vi "WaitForCMD.vi"(0 "Clients ID IN":refnum<k5>[](array[refnum]), 1 "Cmd FIFO IN":T1(array[cluster]), 5 "TCP/IP Error IN":errorcluster, 9 "Excmd VRN":refnum<visa-resource-name>="COM8", 11 "Serial Error IN":errorcluster, 12 "Timeout":u32=25) -> (3 "Cmd FIFO OUT":T1(array[cluster]), 6 "TCP/IP Error":errorcluster, 15 "Serial Error":errorcluster)   [LabVIEW 2019]
panel:
  out "Chaîne":string
  out "ExecTime":u32
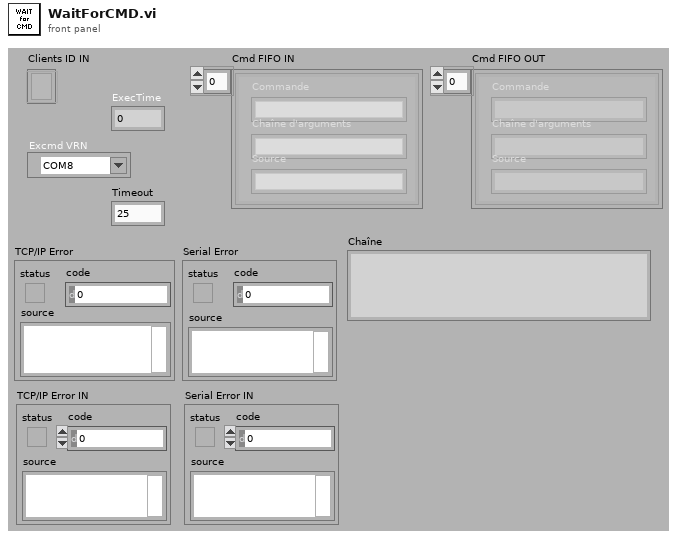
[diagram p1: front panel]
types:
  T1 = cluster{"Commande":string, "Chaîne d'arguments":string, "Source":string}[]
  T2 = cluster{"Commande":string, "data out":string, "Source":string}[]
  T3 = cluster{"Commande":string, "Chaîne":string, "Source":string}[]
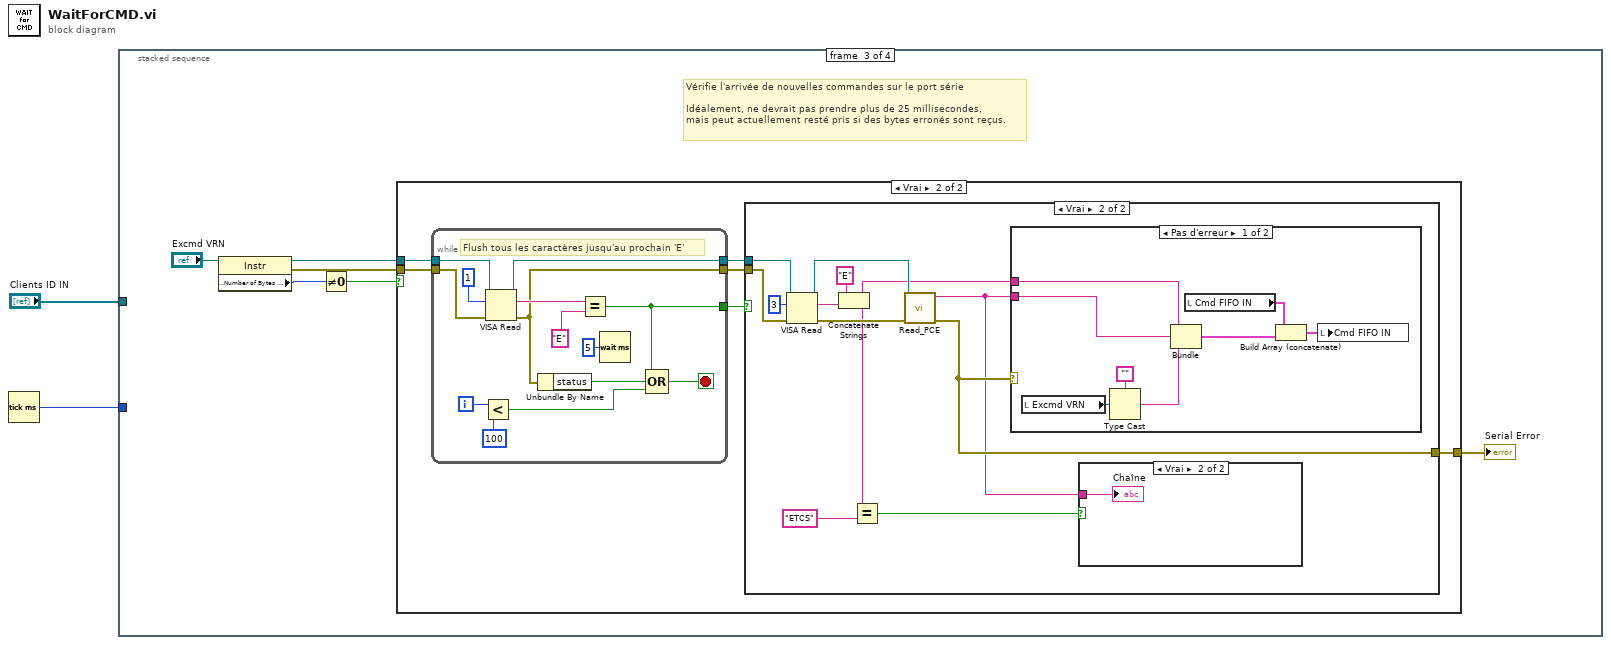
[diagram p0: block diagram]
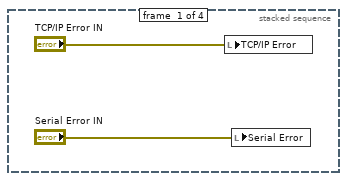
[diagram p2: hidden frame]
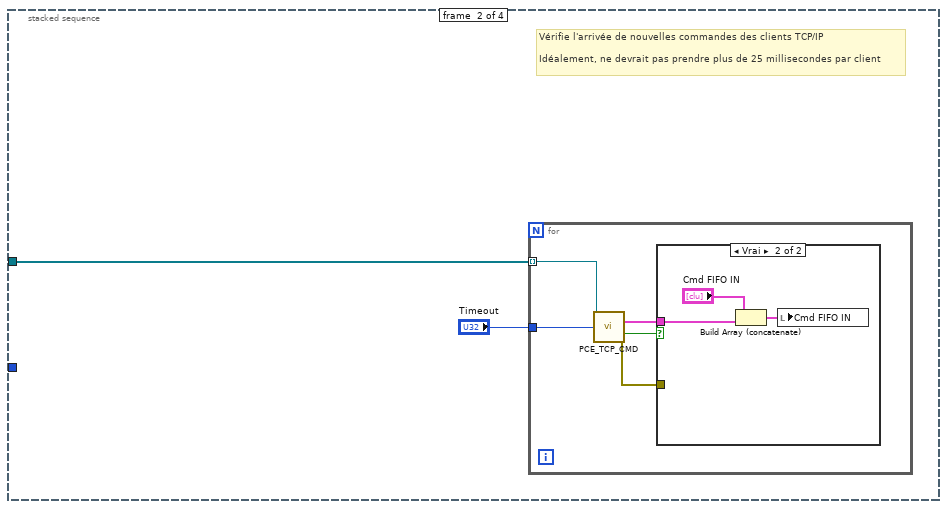
[diagram p3: hidden frame]
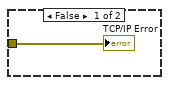
[diagram p4: hidden frame]
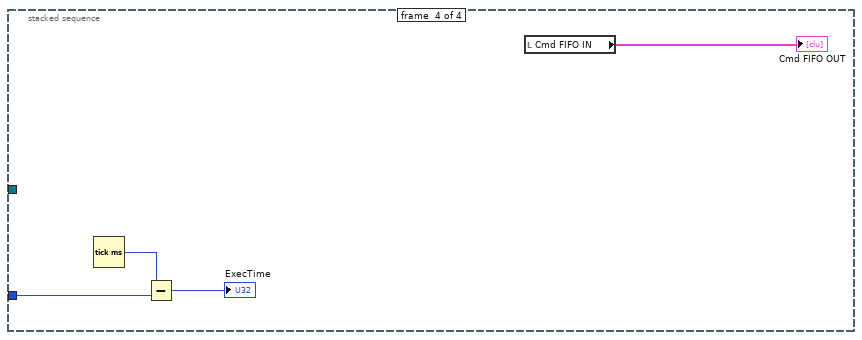
[diagram p9: hidden frame]
diagram:
  n1 = Tick Count (ms)() -> (millisecond timer value=w2:u32)
  n2 = stacked-sequence {
    tunnel: w2 -> [_ _ _ w67]
    tunnel: "Clients ID IN" -> [_ w6 _ _]
    frame #0 {
      n3 = local write "TCP/IP Error"("TCP/IP Error IN") -> ()
      n4 = local write "Serial Error"("Serial Error IN") -> ()
    }
    frame #1 {
      # "Vérifie l'arrivée de nouvelles commandes des clients TCP/IP\n\nIdéalement, ne devrait pas prendre plus de 25 millisecondes par client"
      n5 = for {
        tunnel: w6 -> [w11] mode=indexing
        tunnel: "Timeout" -> [w7]
        n6 = call "PCE_TCP_CMD.vi"("CID IN"=w11, "Timeout"=w7) -> ("FIFOelt"=w9:cluster{string, "data out":string, string}, "Cmd?"=w10:bool, "Error OUT"=w8:errorcluster)  [unwired: 10 in, 1 out]
        n7 = case shown="Vrai" w10 {
          tunnel: w9 -> [_ w14]
          tunnel: w8 -> [w12 _]
          frame False {
            "TCP/IP Error" <- w12
          }
          frame True {
            n8 = Build Array (concatenate)("Cmd FIFO IN", w14) -> (w13:T2)
            n9 = local write "Cmd FIFO IN"(w13) -> ()
          }
        }
      }
    }
    frame #2 {
      # "Vérifie l'arrivée de nouvelles commandes sur le port série\n\nIdéalement, ne devrait pas prendre plus de 25 millisecondes,\nmais peut actuellement resté pris si des bytes erronés sont reçus."
      n10 = property class="Instr"(reference="Excmd VRN") -> (reference out=w19:refnum<visa-resource-name>, error out=w17:errorcluster, "Serial Settings:Number of Bytes at Serial Port"=w20:u32)  [unwired: 1 in]
      n11 = Not Equal To 0?(x=w20) -> (x != 0?=w18:bool)
      n12 = case shown="Vrai" w18 {
        tunnel: w19 -> [_ w28]
        tunnel: w17 -> [w22 w25]
        tunnel: [w22 w23] -> w16
        frame False {
        }
        frame True {
          n13 = while {
            tunnel: [w53] -> w27
            tunnel: w28 -> [w57]
            tunnel: [w56] -> w26
            tunnel: w25 -> [w52]
            tunnel: [w51] -> w24
            i -> [w64]
            stop <- w61 stop-if-true
            # "Flush tous les caractères jusqu'au prochain 'E'"
            n14 = Less?(x=w64, y=100) -> (x < y?=w60:bool)
            n15 = VISA Read(VISA resource name=w57, byte count=u32 1 ("Bytes to Read"), error in (no error)=w52) -> (VISA resource name out=w56:refnum<visa-resource-name>, read buffer=w58:string, error out=w51:errorcluster)  [unwired: 1 out]
            n16 = Unbundle By Name(w51) -> ("status"=w54:bool)
            n17 = Equal?(x=w58, y="E") -> (x = y?=w53:bool)
            n18 = Wait (ms)(milliseconds to wait=u32 5 ("attente (ms)")) -> ()  [unwired: 1 out]
            n19 = Compound Arithmetic op=OR(w53, w54, w60) -> (w61:bool)
          }
          n20 = case shown="Vrai" w27 {
            tunnel: w26 -> [_ w38]
            tunnel: w24 -> [w29 w36]
            tunnel: [w29 w34] -> w23
            frame False {
            }
            frame True {
              n21 = VISA Read(VISA resource name=w38, byte count=u32 3 ("Bytes to Read"), error in (no error)=w36) -> (VISA resource name out=w37:refnum<visa-resource-name>, read buffer=w40:string, error out=w35:errorcluster)  [unwired: 1 out]
              n22 = Concatenate Strings("E", w40) -> (w33:string)
              n23 = Equal?(x=w33, y="ETCS") -> (x = y?=w31:bool)
              n24 = call "Read_PCE.vi"("error in"=w35, "VISA resource name"=w37) -> ("error out"=w34:errorcluster, "Chaîne"=w30:string)  [unwired: 8 in]
              n25 = case shown="Pas d'erreur" w34 {
                tunnel: w30 -> [w45 _]
                tunnel: w33 -> [w46 _]
                frame No Error {
                  n26 = local read "Excmd VRN"() -> (w50:refnum<visa-resource-name>)
                  n27 = Type Cast(type="", x=w50) -> (*(type *) &x=w44:string)
                  n28 = Bundle(w46, "Chaîne"=w45, w44) -> (w43:cluster{string, "Chaîne":string, string})  [unwired: 1 in]
                  n29 = local read "Cmd FIFO IN"() -> (w48:T1)
                  n30 = Build Array (concatenate)(w48, w43) -> (w47:T3)
                  n31 = local write "Cmd FIFO IN"(w47) -> ()
                }
                frame Error {
                }
              }
              n32 = case shown="Vrai" w31 {
                tunnel: w30 -> [_ w42]
                frame False {
                }
                frame True {
                  "Chaîne" <- w42
                }
              }
            }
          }
        }
      }
      "Serial Error" <- w16
    }
    frame #3 {
      n33 = Tick Count (ms)() -> (millisecond timer value=w66:u32)
      n34 = Subtract(x=w66, y=w67) -> (x-y=→"ExecTime":u32)
      n35 = local read "Cmd FIFO IN"() -> (→"Cmd FIFO OUT":T1)
    }
  }
